vi "tsapp_clear_bus_statistics.vi"(8 "error in (no error)":errorcluster caption="错误输入（无错误）", 11 "路径输入":path) -> (0 "error out":errorcluster caption="错误输出", 2 "retuen":i32, 3 "路径输出":path)   [LabVIEW 2014]
doc: "Function Introduction ：\nClear bus statistics data\nCall location ： \ninput parameter ：\nnothing\nReturn value ：\n==0: Execution successfulss\nOther values: Query error code"
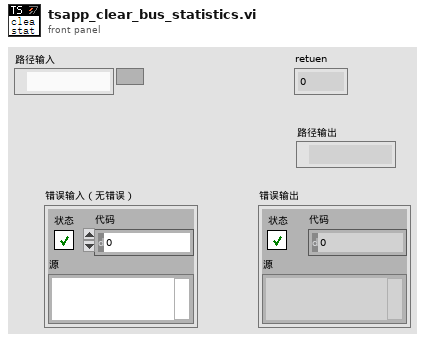
[diagram p1: front panel]
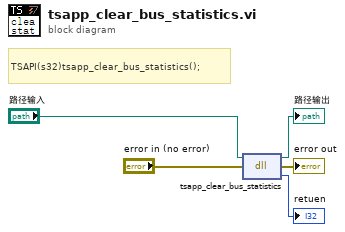
[diagram p0: block diagram]
diagram:
  # "TSAPI(s32)tsapp_clear_bus_statistics();"
  n1 = dll-call lib="D:/Work/LabVIEW Code/TSMaster Labview SDK/LabVIEW/LabVIEW-TSMasterAPI_CLN/TSMasterAPI_LabVIEW-2024-08-02 09-14-06/Not_organized_vi/TSMaster.*" fn="tsapp_clear_bus_statistics"(path in="路径输入", error in="error in (no error)") -> (path out=→"路径输出":path, error out=→"error out":errorcluster, "返回类型"=→"retuen":i32)  [unwired: 1 in]
